vi "LEDprogramMarcoGonzalez.vi"() -> ()   [LabVIEW 2012]
doc: "VI that has 3 Round LEDs on the Front Panel. When you run the program, the first LED should turn on and stay on. After three seconds, the second LED should turn on and stay on. After three more seconds, the third LED should turn on and stay on. All LEDS should be on for 5 more seconds, and then the program ends. Each LED should have a countdown which indicates how much time is left until the next LED comes on."
panel:
  out "Numeric":dbl
  out "Numeric 1":dbl
  out "Tres":bool
  out "Dos":bool
  out "Uno":bool
  # "Marco Gonzalez\nEA3\n03 / 09 /2017"
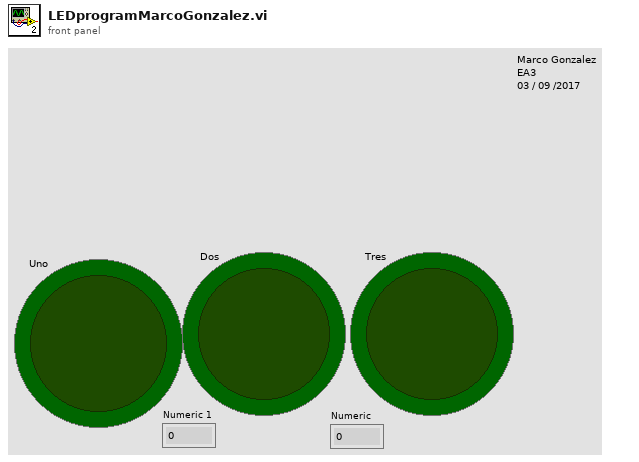
[diagram p1: front panel]
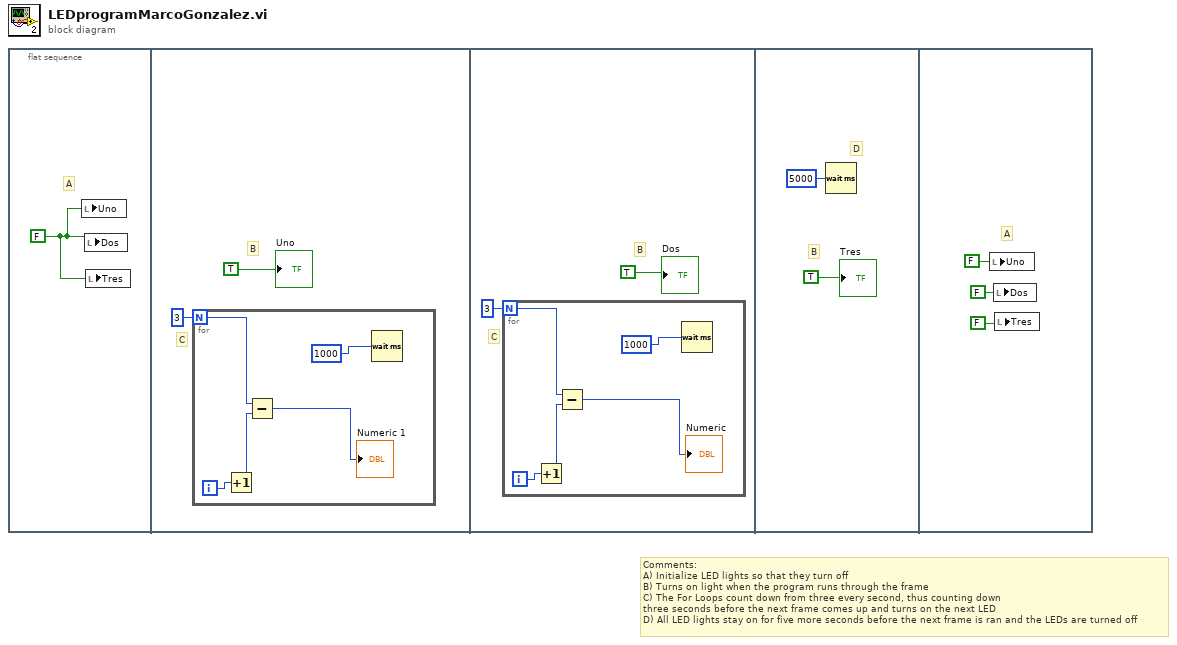
[diagram p0: block diagram]
diagram:
  # "Comments:\nA) Initialize LED lights so that they turn off\nB) Turns on light when the program runs through the frame\nC) The For Loops count down from three every second, thus counting down\nthree seconds before the next frame comes up and turns on the next LED\nD) All LED lights stay on for five more seconds before the next frame is ran and the LEDs are turned off"
  n1 = flat-sequence {
    frame #0 {
      w1 = FALSE
      # "A"
      n2 = local write "Uno"(w1) -> ()
      n3 = local write "Dos"(w1) -> ()
      n4 = local write "Tres"(w1) -> ()
    }
    frame #1 {
      # "C"
      # "B"
      n5 = for {
        N: 3 -> [w5]
        i -> [w7]
        n6 = Increment(x=w7) -> (x+1=w6:i32)
        n7 = Subtract(x=w5, y=w6) -> (x-y=→"Numeric 1":i32)
        n8 = Wait (ms)(milliseconds to wait=u32 1000) -> ()  [unwired: 1 out]
      }
      "Uno" <- TRUE
    }
    frame #2 {
      # "C"
      # "B"
      n9 = for {
        N: 3 -> [w12]
        i -> [w14]
        n10 = Increment(x=w14) -> (x+1=w13:i32)
        n11 = Subtract(x=w12, y=w13) -> (x-y=→"Numeric":i32)
        n12 = Wait (ms)(milliseconds to wait=u32 1000) -> ()  [unwired: 1 out]
      }
      "Dos" <- TRUE
    }
    frame #3 {
      # "D"
      # "B"
      n13 = Wait (ms)(milliseconds to wait=u32 5000) -> ()  [unwired: 1 out]
      "Tres" <- TRUE
    }
    frame #4 {
      # "A"
      n14 = local write "Uno"(FALSE) -> ()
      n15 = local write "Dos"(FALSE) -> ()
      n16 = local write "Tres"(FALSE) -> ()
    }
  }
